vi "ICS425 Read Write.vi"(8 "Error In":errorcluster, 10 "Cmd":string, 11 "VISA (Input)":refnum<visa-resource-name>) -> (0 "Error Out":errorcluster, 2 "read buffer":string, 3 "VISA Refnum (Output)":refnum<visa-resource-name>)   [LabVIEW 2016]
panel:
  out "Serial Settings:Number of Bytes at Serial Port":u32
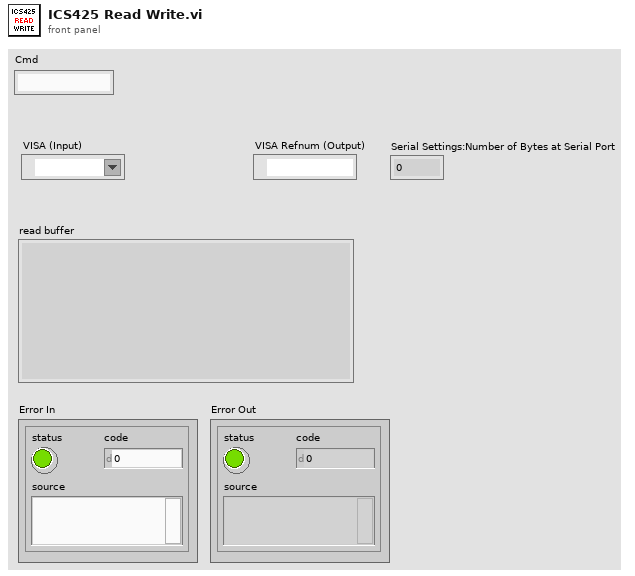
[diagram p1: front panel]
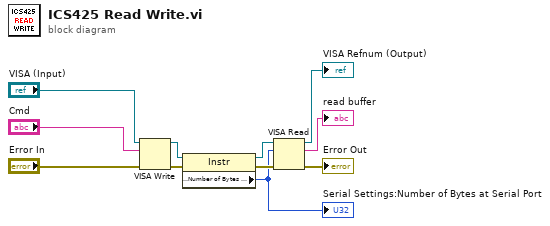
[diagram p0: block diagram]
diagram:
  n1 = VISA Write(VISA resource name="VISA (Input)", write buffer="Cmd", error in (no error)="Error In") -> (VISA resource name out=w9:refnum<visa-resource-name>, error out=w8:errorcluster)  [unwired: 1 out]
  n2 = property class="Instr"(reference=w9, error in=w8) -> (reference out=w6:refnum<visa-resource-name>, error out=w7:errorcluster, "Serial Settings:Number of Bytes at Serial Port"=w5:u32)
  "Serial Settings:Number of Bytes at Serial Port" <- w5
  n3 = VISA Read(VISA resource name=w6, byte count=w5, error in (no error)=w7) -> (VISA resource name out=→"VISA Refnum (Output)":refnum<visa-resource-name>, read buffer=→"read buffer":string, error out=→"Error Out":errorcluster)  [unwired: 1 out]
